vi "ADCP_Processed_Bytes_To_RREQ_Packet.vi"(8 "error in (no error)":errorcluster, 10 "Processed Packet Bytes":u8[](array[numeric]), 11 "ADCP In":refnum<class "ADCP.lvclass">) -> (0 "error out":errorcluster, 2 "RREQ out":T1, 3 "ADCP Out":refnum<class "ADCP.lvclass">)   [LabVIEW 2017, in "ADCP.lvclass"]
uses:
  ADCP.lvclass
  ADCP.lvclass/ADCP.ctl
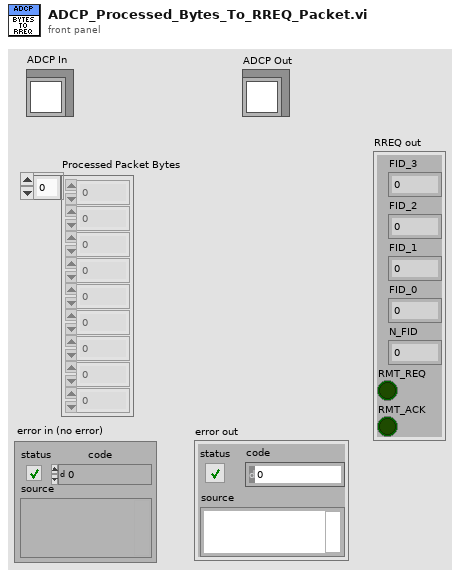
[diagram p1: front panel]
types:
  T1 = cluster{"FID_3":u8, "FID_2":u8, "FID_1":u8, "FID_0":u8, "N_FID":u8, "RMT_REQ":bool, "RMT_ACK":bool}
  T2 = enum16{"Data", "Connection Management", "Remote Request", "Error and status", "INVALID"}
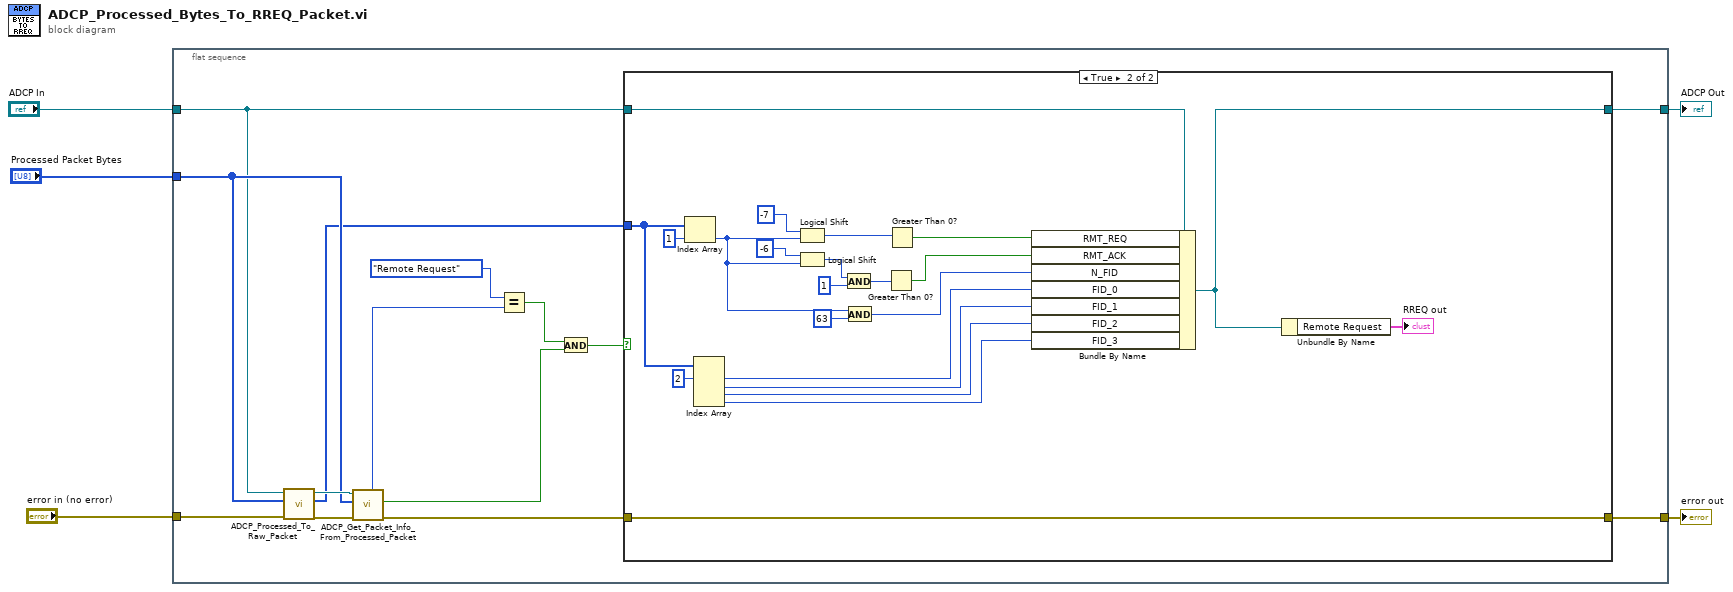
[diagram p0: block diagram]
diagram:
  n1 = flat-sequence {
    tunnel: "ADCP In" -> [w9]
    tunnel: "Processed Packet Bytes" -> [w16]
    tunnel: "error in (no error)" -> [w19]
    tunnel: [w8] -> w2
    tunnel: [w7] -> w1
    frame #0 {
      n2 = call "ADCP_Processed_To_Raw_Packet.vi"("error in (no error)"=w19, "Processed Packet"=w16, "ADCP in"=w9) -> ("error out"=w18:errorcluster, "Raw Packet"=w6:u8[], "ADCP out"=w17:refnum<class "ADCP.lvclass">)  [unwired: 6 in]
      n3 = call "ADCP_Get_Packet_Info_From_Processed_Packet.vi"("error in (no error)"=w18, "Processed Packet"=w16, "ADCP in"=w17) -> ("error out"=w11:errorcluster, "Checksum Valid ?"=w12:bool, "Packet Type"=w15:T2)  [unwired: 2 in, 4 out]
      n4 = Equal?(x=T2."Remote Request", y=w15) -> (x = y?=w13:bool)
      n5 = And(x=w13, y=w12) -> (x .and. y?=w10:bool)
      n6 = case shown="True" w10 {
        tunnel: w11 -> [w21 w31]
        tunnel: [w21 w31] -> w7
        tunnel: w9 -> [w20 w32]
        tunnel: [w20 w23] -> w8
        tunnel: w6 -> [_ w34]
        frame False {
        }
        frame True {
          n7 = Index Array(array=w34, index=1) -> (element=w38:u8)
          n8 = Index Array(array=w34, index #1=2 ("index")) -> (element #1=w27:u8, element #2=w26:u8, element #3=w25:u8, element #4=w24:u8)  [unwired: 3 in]
          n9 = Logical Shift(y=i16 -7, x=w38) -> (x << y=w36:u8)
          n10 = Logical Shift(y=i16 -6, x=w38) -> (x << y=w40:u8)
          n11 = And(x=w40, y=u8 1) -> (x .and. y?=w35:u8)
          n12 = And(x=w38, y=u8 63) -> (x .and. y?=w28:u8)
          n13 = Greater Than 0?(x=w35) -> (x > 0?=w29:bool)
          n14 = Greater Than 0?(x=w36) -> (x > 0?=w30:bool)
          n15 = Bundle By Name(cluster=w32, "RMT_REQ"=w30, "RMT_ACK"=w29, "N_FID"=w28, "FID_0"=w27, "FID_1"=w26, "FID_2"=w25, "FID_3"=w24) -> (w23:refnum<class "ADCP.lvclass">)
          n16 = Unbundle By Name(w23) -> ("Remote Request"=→"RREQ out":T1)
        }
      }
    }
  }
  "ADCP Out" <- w2
  "error out" <- w1
